vi "configure.vi"(8 "error in (no error)":errorcluster, 11 "MG090622IMAQCamera in":refnum<class "DAQ_MG090622Camera.lvclass">) -> (0 "error out":errorcluster, 3 "MG090622IMAQCamera out":refnum<class "DAQ_MG090622Camera.lvclass">)   [LabVIEW 2010, in "DAQ_MG090622Camera.lvclass"]
doc: "The dynamic dispatch version of this VI loads and displays the configuration file associated with the plug-in object. The user modify and save the configuration data."
uses:
  DAQ_MG090622Camera.lvclass
  common/classes/GenericComponent/GenericComponent/GenericComponent.lvclass
  common/classes/ErrorController/ErrorController/ErrorController.lvclass
  camera_type_enum.ctl
  connection_type_enum.ctl
panel:
  in  "Tab Control":enum32{"Description", "Device"}(tab)
  in  "Device name":string
  in  "camera type":T1
  in  "connection type":T2=enum."USB"
  out "Configuration":string
  in  "cancel button":bool
  in  "save button":bool
  # "Configure DAQ_MG090622Camera"
  # "The DAQ_MG09622Camera component encapsulates as a camera device assible via the National Instruments IMAQ interface."
  # "... as specified in Measurement & Automation Explorer"
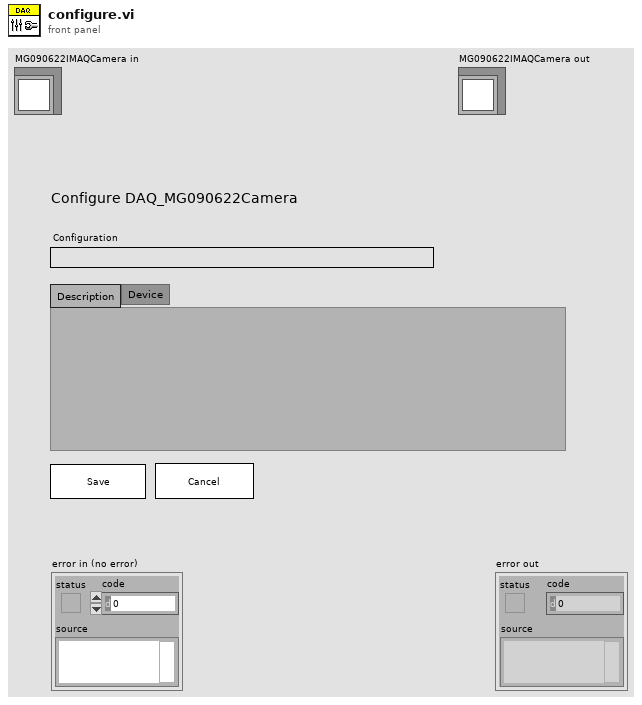
[diagram p1: front panel]
types:
  T1 = typedef "DAQ_MG090622Camera.lvclass/camera_type_enum.ctl" = enum16{"gray scale", "RGB"}
  T2 = typedef "DAQ_MG090622Camera.lvclass/connection_type_enum.ctl" = enum16{"IEEE 1394 (FireWire)", "USB", "GigE", "CameraLink"}
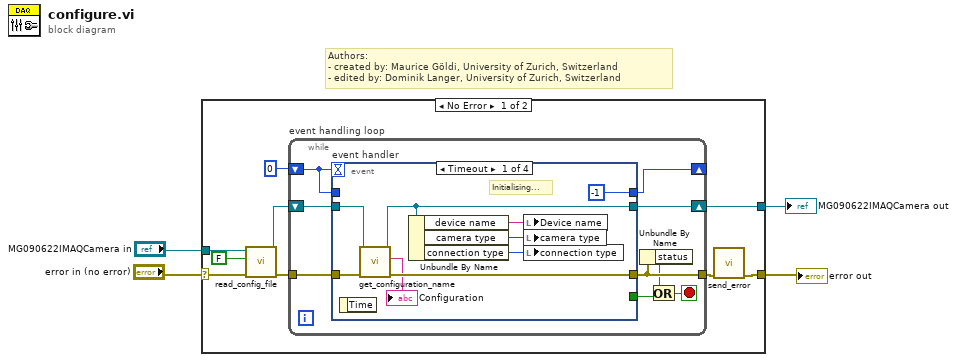
[diagram p0: block diagram]
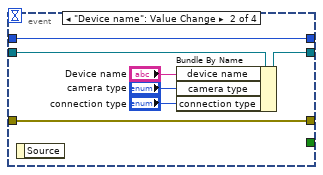
[diagram p2: hidden frame]
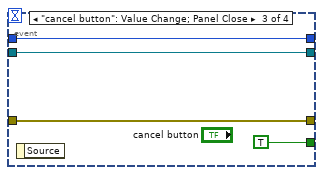
[diagram p3: hidden frame]
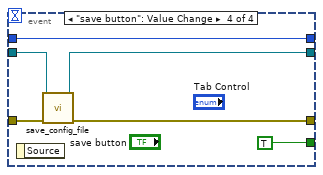
[diagram p4: hidden frame]
diagram:
  # "Authors: \n- created by: Maurice Göldi, University of Zurich, Switzerland\n- edited by: Dominik Langer, University of Zurich, Switzerland"
  n1 = case shown="No Error" "error in (no error)" {
    selector: "error in (no error)" -> [w13 w50]
    tunnel: "MG090622IMAQCamera in" -> [w12 w49]
    tunnel: [w6 w50] -> w2
    tunnel: [w7 w49] -> w1
    frame No Error {
      n2 = call-dynamic "read_config_file.vi"("error in (no error)"=w13, "force load?"=FALSE, "GenericPlugin in"=w12) -> ("error out"=w10:errorcluster, "GenericPlugin out"=w8:refnum<class "DAQ_MG090622Camera.lvclass">)  [unwired: 7 out]
      n3 = while "event handling loop" {
        shift-right: [w20] -> _
        shift-left: 0 -> [w21]
        shift-right: [w18] -> w7
        shift-left: w8 -> [w19]
        tunnel: w10 -> [w22]
        tunnel: [w17] -> w5
        stop <- w14 stop-if-true
        n4 = event "event handler" shown="[0] Timeout" {
          selector: _ -> [_ _ _ _]
          dyn-events: _ -> [_ _ _ _]
          timeout: w21 -> [_ _ _ _]
          tunnel: w22 -> [w28 w38 w40 w47]
          tunnel: [w25 w38 w40 w46] -> w17
          tunnel: [-1 w37 w42 w48] -> w20
          tunnel: w21 -> [_ w37 w42 w48]
          tunnel: w19 -> [w27 w35 w41 w43]
          tunnel: [w26 w34 w41 w45] -> w18
          tunnel: [_ _ TRUE TRUE] -> w16
          event Timeout {
            # "Initialising..."
            n5 = event-data() -> ()  [unwired: 2 out]
            n6 = call "get_configuration_name.vi"("error in (no error)"=w28, "GenericPlugin.lvclass in"=w27) -> ("error out"=w25:errorcluster, "configuration name"=→"Configuration":string, "GenericPlugin.lvclass out"=w26:refnum<class "DAQ_MG090622Camera.lvclass">)  [unwired: 7 in]
            n7 = Unbundle By Name(w26) -> ("device name"=w30:string, "camera type"=w29:T1, "connection type"=w23:T2)
            n8 = local write "Device name"(w30) -> ()
            n9 = local write "camera type"(w29) -> ()
            n10 = local write "connection type"(w23) -> ()
          }
          event "Device name": Value Change {
            n11 = event-data() -> ()  [unwired: 2 out]
            n12 = Bundle By Name(cluster=w35, "device name"="Device name", "camera type"="camera type", "connection type"="connection type") -> (w34:refnum<class "DAQ_MG090622Camera.lvclass">)
          }
          event "cancel button": Value Change; Panel Close {
            n13 = event-data() -> ()  [unwired: 2 out]
          }
          event "save button": Value Change {
            n14 = event-data() -> ()  [unwired: 2 out]
            n15 = call-dynamic "save_config_file.vi"("error in (no error)"=w47, "GenericPlugin in"=w43) -> ("error out"=w46:errorcluster, "GenericPlugin out"=w45:refnum<class "DAQ_MG090622Camera.lvclass">)  [unwired: 1 in, 7 out]
          }
        }
        n16 = Unbundle By Name(w17) -> ("status"=w15:bool)
        n17 = Or(x=w15, y=w16) -> (x .or. y?=w14:bool)
      }
      n18 = call "send_error.vi"("error in (no error)"=w5) -> ("error out"=w6:errorcluster)  [unwired: 10 in]
    }
    frame Error {
    }
  }
  "error out" <- w2
  "MG090622IMAQCamera out" <- w1
